vi "Line Detector Create rusin_dat.vi"(8 "Error In":errorcluster, 9 "header":string, 10 "Initial fit guess":dbl[][](array[numeric]) format="%#_4p", 11 "File Path Control":path) -> (0 "Error Out":errorcluster)   [LabVIEW 2016]
panel:
  # "F0         dF     Ampl   Phase   Xbgrd   Ybgrd"
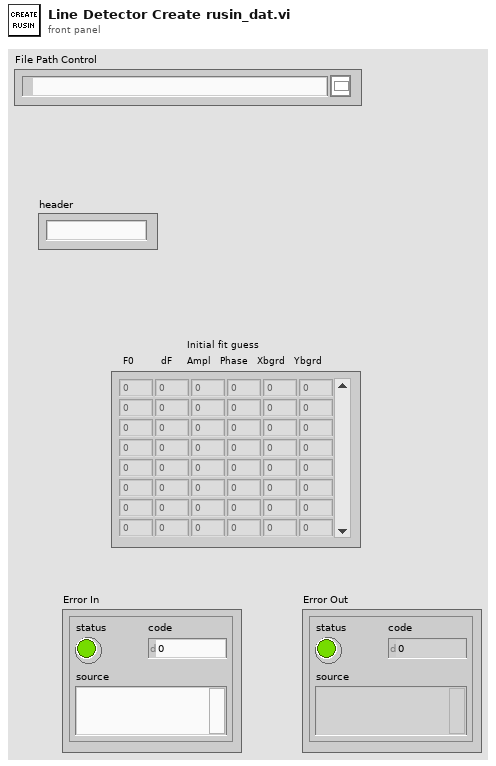
[diagram p1: front panel]
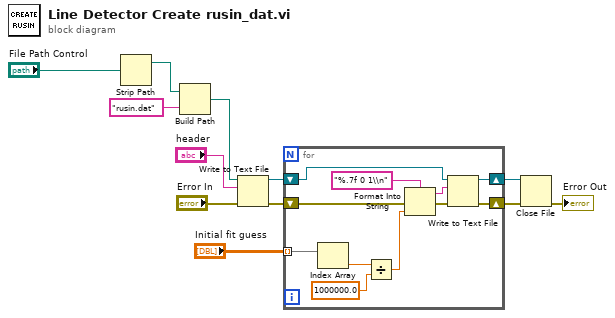
[diagram p0: block diagram]
diagram:
  n1 = Strip Path(path="File Path Control") -> (stripped path=w9:path)  [unwired: 1 out]
  n2 = Build Path(base path=w9, name or relative path="rusin.dat") -> (appended path=w7:path)
  n3 = Write to Text File(file (use dialog)=w7, text="header", error in="Error In") -> (refnum out=w6:refnum<file>, error out=w5:errorcluster)  [unwired: 1 in, 1 out]
  n4 = for {
    tunnel: "Initial fit guess" -> [w21] mode=indexing
    shift-right: [w14] -> w4
    shift-left: w5 -> [w15]
    shift-right: [w13] -> w3
    shift-left: w6 -> [w23]
    n5 = Index Array(array=w21) -> (element=w22:dbl)  [unwired: 1 in]
    n6 = Divide(x=w22, y=1000000.0) -> (x/y=w19:dbl)
    n7 = Format Into String(format string="%.7f 0 1\\n", error in=w15, w19) -> (resulting string=w17:string, error out=w16:errorcluster)  [unwired: 1 in]
    n8 = Write to Text File(file (use dialog)=w23, text=w17, error in=w16) -> (refnum out=w13:refnum<file>, error out=w14:errorcluster)  [unwired: 1 in, 1 out]
  }
  n9 = Close File(refnum=w3, error in=w4) -> (error out=→"Error Out":errorcluster)  [unwired: 1 out]
